vi "Read IO Configuration File.vi"(8 "error in (no error)":errorcluster, 11 "DAQ ConfigFile":path) -> (0 "error out":errorcluster, 1 "default file created":bool, 2 "IO Nodes":T2={"DI Config"={"DI Tasks"=[]}, "DO Config"={"DO Channels"=[{"DevName"="Mod5-9482-SIM", "IOName"="", "IOPath"="Mod5-9482-SIM/port0/line0", "SchemName"="CH0", "logic"=enum."Hi", "DAQmx Task"=""}, {"DevName"="Mod5-9482-SIM", "IOName"="", "IOPath"="Mod5-9482-SIM/port0/line1", "SchemName"="CH1", "logic"=enum."Hi", "DAQmx Task"=""}, {"DevName"="Mod5-9482-SIM", "IOName"="", "IOPath"="Mod5-9482-SIM/port0/line2", "SchemName"="CH2", "logic"=enum."Hi", "DAQmx Task"=""}, {"DevName"="Mod5-9482-SIM", "IOName"="", "IOPath"="Mod5-9482-SIM/port0/line3", "SchemName"="CH3", "logic"=enum."Hi", "DAQmx Task"=""}]}, "AI Config"={"AI Tasks"=[{"AI TaskName"="Mod1-9225-SIM", "AI Channels"=[]}, {"AI TaskName"="Mod1-9225-SIM", "AI Channels"=[]}, {"AI TaskName"="Mod1-9225-SIM", "AI Channels"=[]}, {"AI TaskName"="Mod2-9227-SIM", "AI Channels"=[]}, {"AI TaskName"="Mod2-9227-SIM", "AI Channels"=[]}, {"AI TaskName"="Mod4-9205-SIM", "AI Channels"=[]}]}, "AO Config"={"AO Channels"=[{"DevName"="Mod3-9263-SIM", "IOName"="", "IOPath"="Mod3-9263-SIM/ao0", "SchemName"="9263AO0", "Vmin"=-10.0, "Vmax"=10.0, "Conversion"={"MaxSignal"=10.0, "MinSignal"=0.0, "MaxEngUnit"=10.0, "MinEngUnit"=0.0, "ScaleOffset"=0.0, "negate"=FALSE}, "DAQmx Task"=""}]}} {"AO Config"."AO Channels"."Conversion"."ScaleOffset" format="%.3f"; "AO Config"."AO Channels"."Conversion"."MinEngUnit" format="%.3f"; "AO Config"."AO Channels"."Conversion"."MaxEngUnit" format="%.3f"; "AO Config"."AO Channels"."Conversion"."MinSignal" format="%.3f"; "AO Config"."AO Channels"."Conversion"."MaxSignal" format="%.3f"; "AI Config"."AI Tasks"."AI Channels"."Conversion"."ScaleOffset" format="%.3f"; "AI Config"."AI Tasks"."AI Channels"."Conversion"."MinEngUnit" format="%.3f"; "AI Config"."AI Tasks"."AI Channels"."Conversion"."MaxEngUnit" format="%.3f"; "AI Config"."AI Tasks"."AI Channels"."Conversion"."MinSignal" format="%.3f"; "AI Config"."AI Tasks"."AI Channels"."Conversion"."MaxSignal" format="%.3f"; "AI Config"."AI Tasks"."AI Channels"."Terminal Configuration" items=["default"=-1, "RSE"=10083, "NRSE"=10078, "Differential"=10106, "Pseudodifferential"=12529]}, 3 "ConfigFolder out":path, 5 "offsets":T1)   [LabVIEW 2022 SP3, in "DAQ.lvclass"]
doc: "Developed by Kevin Thompson\nkevin@thompsonengineering.net\n\nCopyright 2015\nThompson Engineering, LLC\nReads file: \"IOConfig.ini\" at \"ConfigFolder\" folder."
uses:
  DAQ.lvclass
  DataTypes/TD IO Node Definition--cluster.ctl
  DataTypes/TD DI Config--cluster.ctl
  DataTypes/TD DI Task--cluster.ctl
  DataTypes/TD DI Channel--cluster.ctl
  DataTypes/TD DO Config--cluster.ctl
  DataTypes/TD DO Channel--cluster.ctl
  DataTypes/TD AI Config--cluster.ctl
  DataTypes/TD AI Task--cluster.ctl
  DataTypes/TD AI Channel--cluster.ctl
  DataTypes/TD DataValueConversion--cluster.ctl
  DataTypes/TD AI DAQ Type--enum.ctl
  DataTypes/TD AI Force Bridge--cluster.ctl
  DataTypes/TD AO Config--cluster.ctl
  DataTypes/TD AO Channel--cluster.ctl
  DataTypes/offsets cluster.ctl
  <userlib>/_OpenG.lib/file/file.llb/File Exists - Scalar__ogtk.vi
  DAQ.lvclass/DAQ.ctl
panel:
  # "Reads file: \"IOConfig.ini\"\nat \"ConfigFolder\" folder."
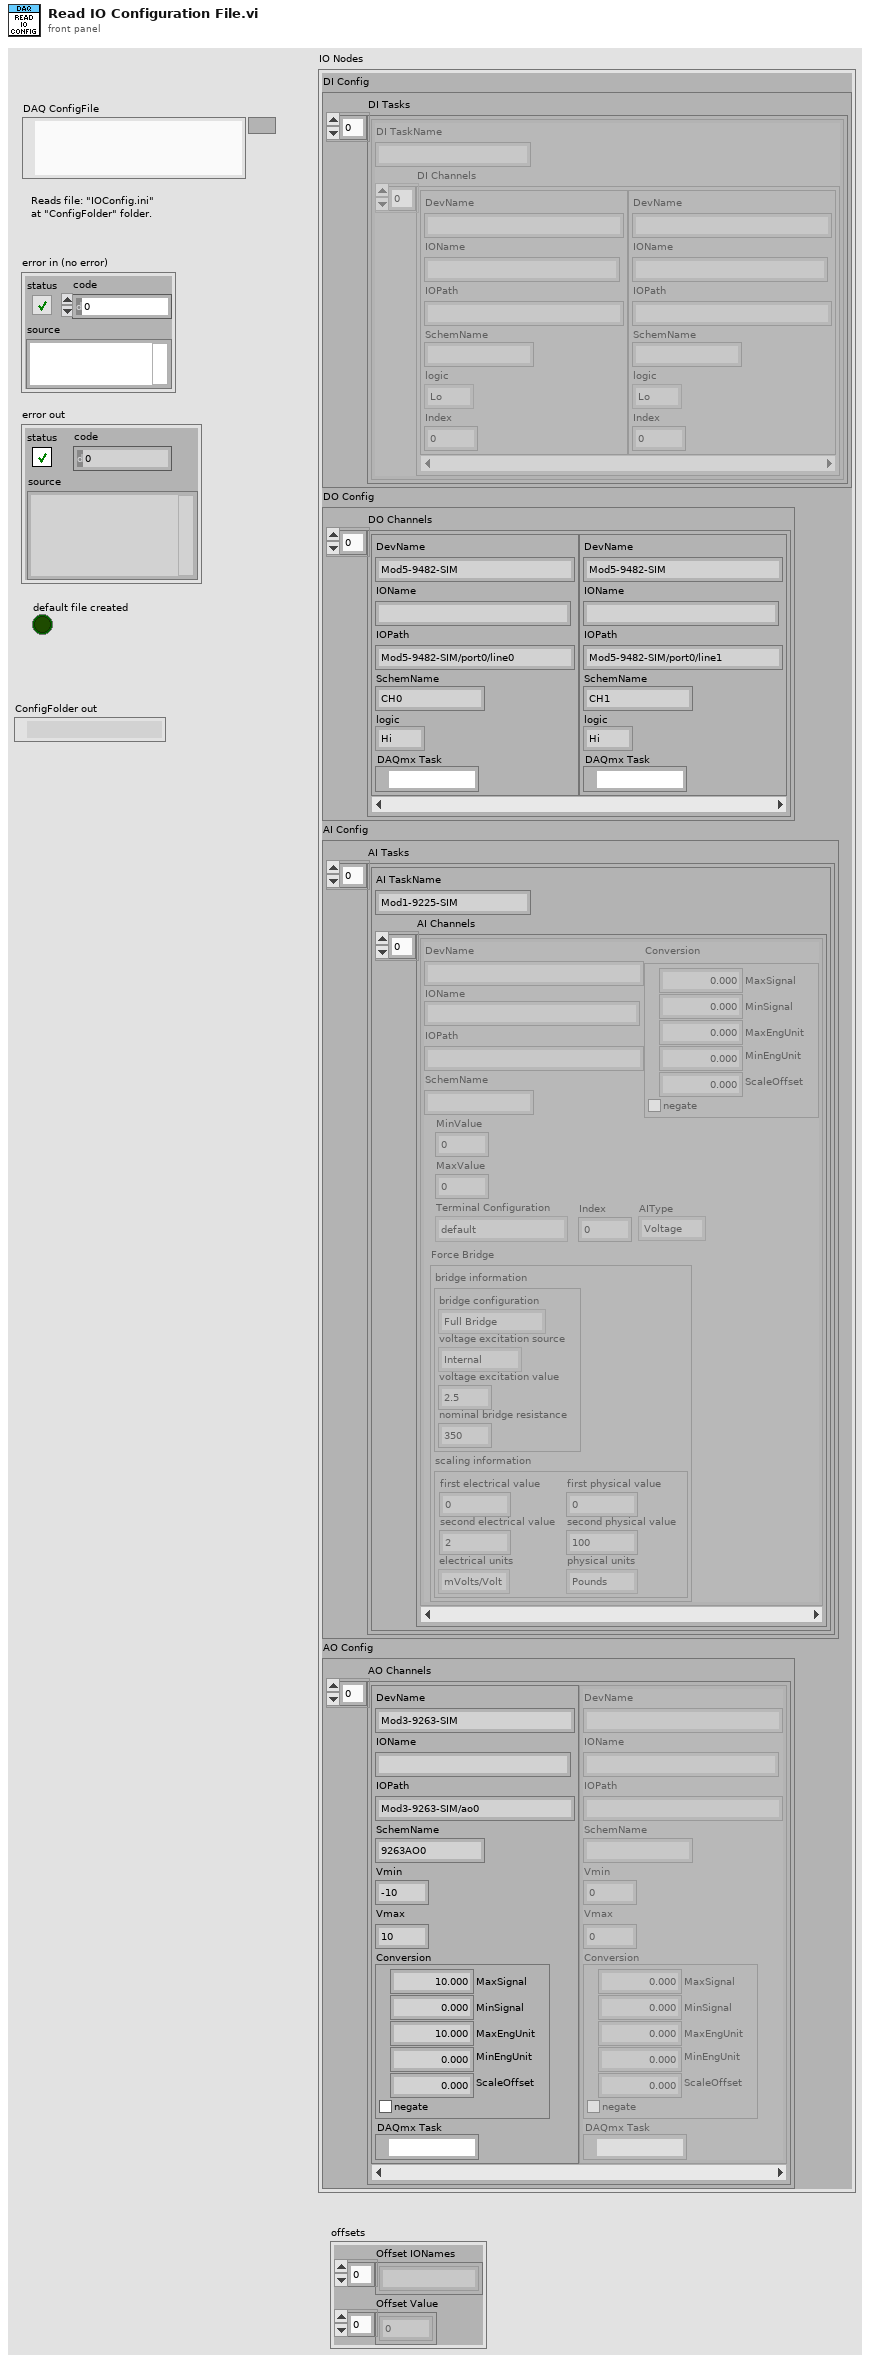
[diagram p1: front panel]
types:
  T1 = typedef "DAQ.lvclass/offsets cluster.ctl" = cluster{"Offset IONames":string[], "Offset Value":dbl[]}
  T2 = typedef "DAQ.lvclass/TD IO Node Definition--cluster.ctl" = cluster{"DI Config":T3, "DO Config":T6, "AI Config":T8, "AO Config":T14}
  T3 = typedef "DAQ.lvclass/TD DI Config--cluster.ctl" = cluster{"DI Tasks":T4[]}
  T4 = typedef "DAQ.lvclass/TD DI Task--cluster.ctl" = cluster{"DI TaskName":string, "DI Channels":T5[]}
  T5 = typedef "DAQ.lvclass/TD DI Channel--cluster.ctl" = cluster{"DevName":string, "IOName":string, "IOPath":string, "SchemName":string, "logic":enum16{"Lo", "Hi"}, "Index":i32}
  T6 = typedef "DAQ.lvclass/TD DO Config--cluster.ctl" = cluster{"DO Channels":T7[]}
  T7 = typedef "DAQ.lvclass/TD DO Channel--cluster.ctl" = cluster{"DevName":string, "IOName":string, "IOPath":string, "SchemName":string, "logic":enum16{"Lo", "Hi"}, "DAQmx Task":refnum<k21>}
  T8 = typedef "DAQ.lvclass/TD AI Config--cluster.ctl" = cluster{"AI Tasks":T9[]}
  T9 = typedef "DAQ.lvclass/TD AI Task--cluster.ctl" = cluster{"AI TaskName":string, "AI Channels":T10[]}
  T10 = typedef "DAQ.lvclass/TD AI Channel--cluster.ctl" = cluster{"DevName":string, "IOName":string, "IOPath":string, "SchemName":string, "MinValue":dbl, "MaxValue":dbl, "Terminal Configuration":i32, "Index":i32, "Conversion":T11, "AIType":T12, "Force Bridge":T13}
  T11 = typedef "DAQ.lvclass/TD DataValueConversion--cluster.ctl" = cluster{"MaxSignal":dbl, "MinSignal":dbl, "MaxEngUnit":dbl, "MinEngUnit":dbl, "ScaleOffset":dbl, "negate":bool}
  T12 = typedef "DAQ.lvclass/TD AI DAQ Type--enum.ctl" = enum16{"Voltage", "Current", "Strain Gage", "Force Bridge"}
  T13 = typedef "DAQ.lvclass/TD AI Force Bridge--cluster.ctl" = cluster{"bridge information":cluster{"bridge configuration":i32, "voltage excitation source":i32, "voltage excitation value":dbl, "nominal bridge resistance":dbl}, "scaling information":cluster{"first electrical value":dbl, "second electrical value":dbl, "electrical units":i32, "first physical value":dbl, "second physical value":dbl, "physical units":i32}}
  T14 = typedef "DAQ.lvclass/TD AO Config--cluster.ctl" = cluster{"AO Channels":T15[]}
  T15 = typedef "DAQ.lvclass/TD AO Channel--cluster.ctl" = cluster{"DevName":string, "IOName":string, "IOPath":string, "SchemName":string, "Vmin":dbl, "Vmax":dbl, "Conversion":T11, "DAQmx Task":refnum<k21>}
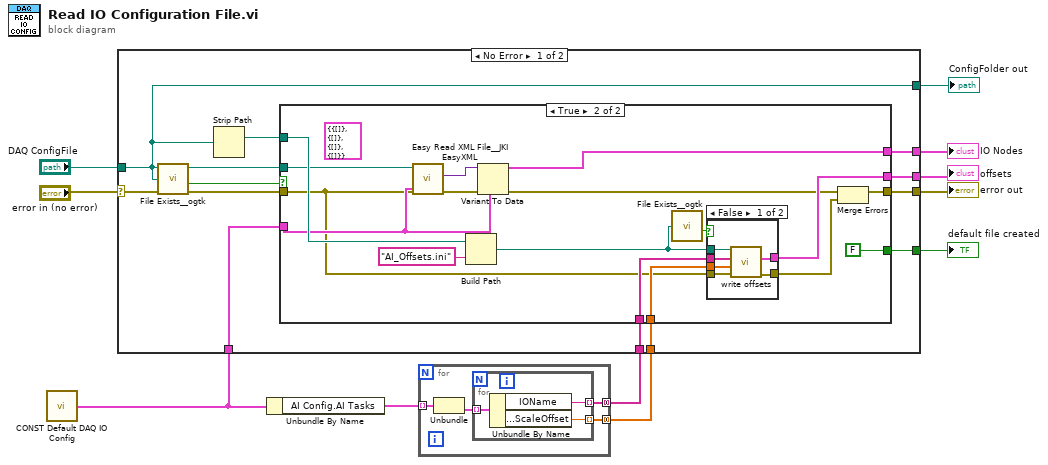
[diagram p0: block diagram]
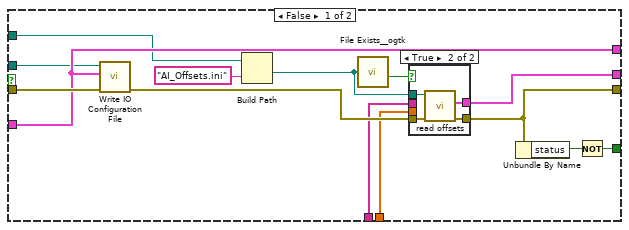
[diagram p2: hidden frame]
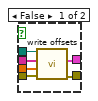
[diagram p3: hidden frame]
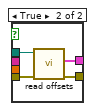
[diagram p4: hidden frame]
diagram:
  n1 = call "CONST Default DAQ IO Config.vi"() -> ("IO Nodes"=w1:T2)  [unwired: 1 in]
  n2 = Unbundle By Name(w1) -> ("AI Config.AI Tasks"=w4:T9[])
  n3 = for {
    tunnel: w4 -> [w15] mode=indexing
    tunnel: [w13] -> w3 mode=concatenating
    tunnel: [w12] -> w2 mode=concatenating
    n4 = Unbundle(w15) -> ("AI Channels"=w14:T10[])  [unwired: 1 out]
    n5 = for {
      tunnel: [w18] -> w13 mode=indexing
      tunnel: [w17] -> w12 mode=indexing
      tunnel: w14 -> [w16] mode=indexing
      n6 = Unbundle By Name(w16) -> ("IOName"=w18:string, "Conversion.ScaleOffset"=w17:dbl)
    }
  }
  n7 = case shown="No Error" "error in (no error)" {
    selector: "error in (no error)" -> [w27 w82]
    tunnel: "DAQ ConfigFile" -> [w19 w81]
    tunnel: [w29 _] -> w11
    tunnel: [w28 w82] -> w6
    tunnel: [w25 _] -> w9
    tunnel: [w19 w81] -> w8
    tunnel: w1 -> [w24 _]
    tunnel: [w23 _] -> w5
    tunnel: w3 -> [w22 _]
    tunnel: w2 -> [w21 _]
    frame No Error {
      n8 = call-poly <userlib>:"File Exists__ogtk.vi"("file path"=w19) -> ("exists"=w26:bool)  [unwired: 6 in, 1 out]
      n9 = Strip Path(path=w19) -> (stripped path=w20:path)  [unwired: 1 out]
      n10 = case shown="True" w26 {
        tunnel: w19 -> [w39 w57]
        tunnel: [w42 w54] -> w29
        tunnel: [w34 w68] -> w28
        tunnel: w27 -> [w43 w56]
        tunnel: w20 -> [w37 w66]
        tunnel: w24 -> [w42 w58]
        tunnel: [w40 FALSE] -> w25
        tunnel: [w35 w69] -> w23
        tunnel: w22 -> [w31 w62]
        tunnel: w21 -> [w30 w61]
        frame False {
          n11 = call "Write IO Configuration File.vi"("error in (no error)"=w43, "IO Nodes"=w42, "DAQ ConfigFile"=w39) -> ("error out"=w33:errorcluster)  [unwired: 8 in]
          n12 = Build Path(base path=w37, name or relative path="AI_Offsets.ini") -> (appended path=w32:path)
          n13 = call-poly <userlib>:"File Exists__ogtk.vi"("file path"=w32) -> ("exists"=w36:bool)  [unwired: 6 in, 1 out]
          n14 = case shown="True" w36 {
            tunnel: [w47 w53] -> w35
            tunnel: w33 -> [w49 w52]
            tunnel: [w48 w51] -> w34
            tunnel: w32 -> [w44 w50]
            tunnel: w31 -> [w46 _]
            tunnel: w30 -> [w45 _]
            frame False {
              n15 = call "write offsets.vi"("error in (no error)"=w49, "Offset Value"=w45, "Offset IOName"=w46, "offsets.ini file"=w44) -> ("error out"=w48:errorcluster, "offsets"=w47:T1)  [unwired: 6 in]
            }
            frame True {
              n16 = call "read offsets.vi"("error in (no error)"=w52, "offsets.ini path"=w50) -> ("error out"=w51:errorcluster, "offsets"=w53:T1)  [unwired: 8 in]
            }
          }
          n17 = Unbundle By Name(w34) -> ("status"=w41:bool)
          n18 = Not(x=w41) -> (.not. x?=w40:bool)
        }
        frame True {
          (unwired) T2 {"DI Config"={"DI Tasks"=[]}, "DO Config"={"DO Channels"=[]}, "AI Config"={"AI Tasks"=[]}, "AO Config"={"AO Channels"=[]}} ("IO Nodes")
          n19 = call <vilib>:"Easy Read XML File__JKI EasyXML.vi"("error in (no error)"=w56, "LabVIEW Data (Type)"=w58, "XML File Path"=w57) -> ("error out"=w59:errorcluster, "LabVIEW Data"=w60:variant)  [unwired: 6 in, 1 out]
          n20 = Build Path(base path=w66, name or relative path="AI_Offsets.ini") -> (appended path=w64:path)
          n21 = Variant To Data(error in=w59, type=w58, Variant=w60) -> (data=w54:T2, error out=w55:errorcluster)
          n22 = call-poly <userlib>:"File Exists__ogtk.vi"("file path"=w64) -> ("exists"=w63:bool)  [unwired: 6 in, 1 out]
          n23 = case shown="False" w63 {
            tunnel: [w74 w80] -> w69
            tunnel: w56 -> [w76 w79]
            tunnel: [w75 w78] -> w67
            tunnel: w64 -> [w71 w77]
            tunnel: w62 -> [w73 _]
            tunnel: w61 -> [w72 _]
            frame False {
              n24 = call "write offsets.vi"("error in (no error)"=w76, "Offset Value"=w72, "Offset IOName"=w73, "offsets.ini file"=w71) -> ("error out"=w75:errorcluster, "offsets"=w74:T1)  [unwired: 6 in]
            }
            frame True {
              n25 = call "read offsets.vi"("error in (no error)"=w79, "offsets.ini path"=w77) -> ("error out"=w78:errorcluster, "offsets"=w80:T1)  [unwired: 8 in]
            }
          }
          n26 = Merge Errors(w55, w67) -> (w68:errorcluster)
        }
      }
    }
    frame Error {
    }
  }
  "IO Nodes" <- w11
  "error out" <- w6
  "default file created" <- w9
  "ConfigFolder out" <- w8
  "offsets" <- w5
